vi "Score Gear Auto.vi"(8 "Command Info in":T1, 9 "speed of backing up":dbl=0.3 format="%#_13g", 10 "Seconds of backing up":dbl=2.0 format="%#_13g") -> (0 "Command Info Out":T1)   [LabVIEW 2016]
uses:
  <vilib>/Rock Robotics/WPI/Framework/Command Status Info.ctl
  <vilib>/Rock Robotics/WPI/Framework/Completion Status.ctl
  <vilib>/Rock Robotics/WPI/Framework/Completion Notifier.ctl
  <vilib>/Rock Robotics/WPI/Solenoid/WPI_SolenoidValue.ctl
  <vilib>/Rock Robotics/WPI/Solenoid/WPI_SolenoidSetEnum.vi
panel:
  in  "Seconds to wait 2":dbl=0.25 format="%#_13g"
  in  "Seconds to wait":dbl=0.15 format="%#_13g"
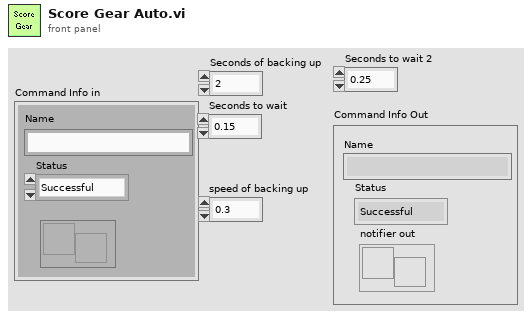
[diagram p1: front panel]
types:
  T1 = typedef "Command Status Info.ctl" = cluster{"Name":string, "Status":T2, "notifier out":T3}
  T2 = typedef "Completion Status.ctl" = enum16{"Successful", "Aborted", "Incomplete"}
  T3 = typedef "Completion Notifier.ctl" = refnum<notifier>
  T4 = typedef "WPI_SolenoidValue.ctl" = enum16{"Off", "On", "Forward", "Reverse"}
  T5 = typedef "WPI_MotorControlDeviceRef.ctl" = cluster{"DeviceStatus":errorcluster, "Type":T6, "PWM":cluster{"PWM Channel":T7, "DeadBand":T8}, "CAN":cluster{"Device Number":u8, "SetOutput VI Ref":variant, "GetOutput VI Ref":variant, "Enable VI Ref":variant, "Disable VI Ref":variant, "Data":variant}, "Invert":bool}
  T6 = typedef "WPI_MotorControlType.ctl" = enum16{"PWM", "CAN"}
  T7 = typedef "FPGA_DIOPWMChannel.ctl" = enum8{"PWM 0", "PWM 1", "PWM 2", "PWM 3", "PWM 4", "PWM 5", "PWM 6", "PWM 7", "PWM 8", "PWM 9", "PWM MXP 0", "PWM MXP 1", "PWM MXP 2", "PWM MXP 3", "PWM MXP 4", "PWM MXP 5", "PWM MXP 6", "PWM MXP 7", "PWM MXP 8", "PWM MXP 9", "Invalid"}
  T8 = typedef "WPI_PWMDeadband.ctl" = cluster{"Name":string, "maxPositivePwm":i32, "minPositivePwm":i32, "centerPwm":i32, "maxNegativePwm":i32, "minNegativePwm":i32, "angularRange":u16}
  T9 = typedef "WPI_SolenoidDevRef.ctl" = cluster{"DevStatus":errorcluster, "Pneumatics Control Module":u8, "Forward Solenoid Channel":T10, "Reverse Solenoid Channel":T10}
  T10 = typedef "WPI_SolenoidChannel.ctl" = enum8{"Solenoid 0", "Solenoid 1", "Solenoid 2", "Solenoid 3", "Solenoid 4", "Solenoid 5", "Solenoid 6", "Solenoid 7", "Invalid"}
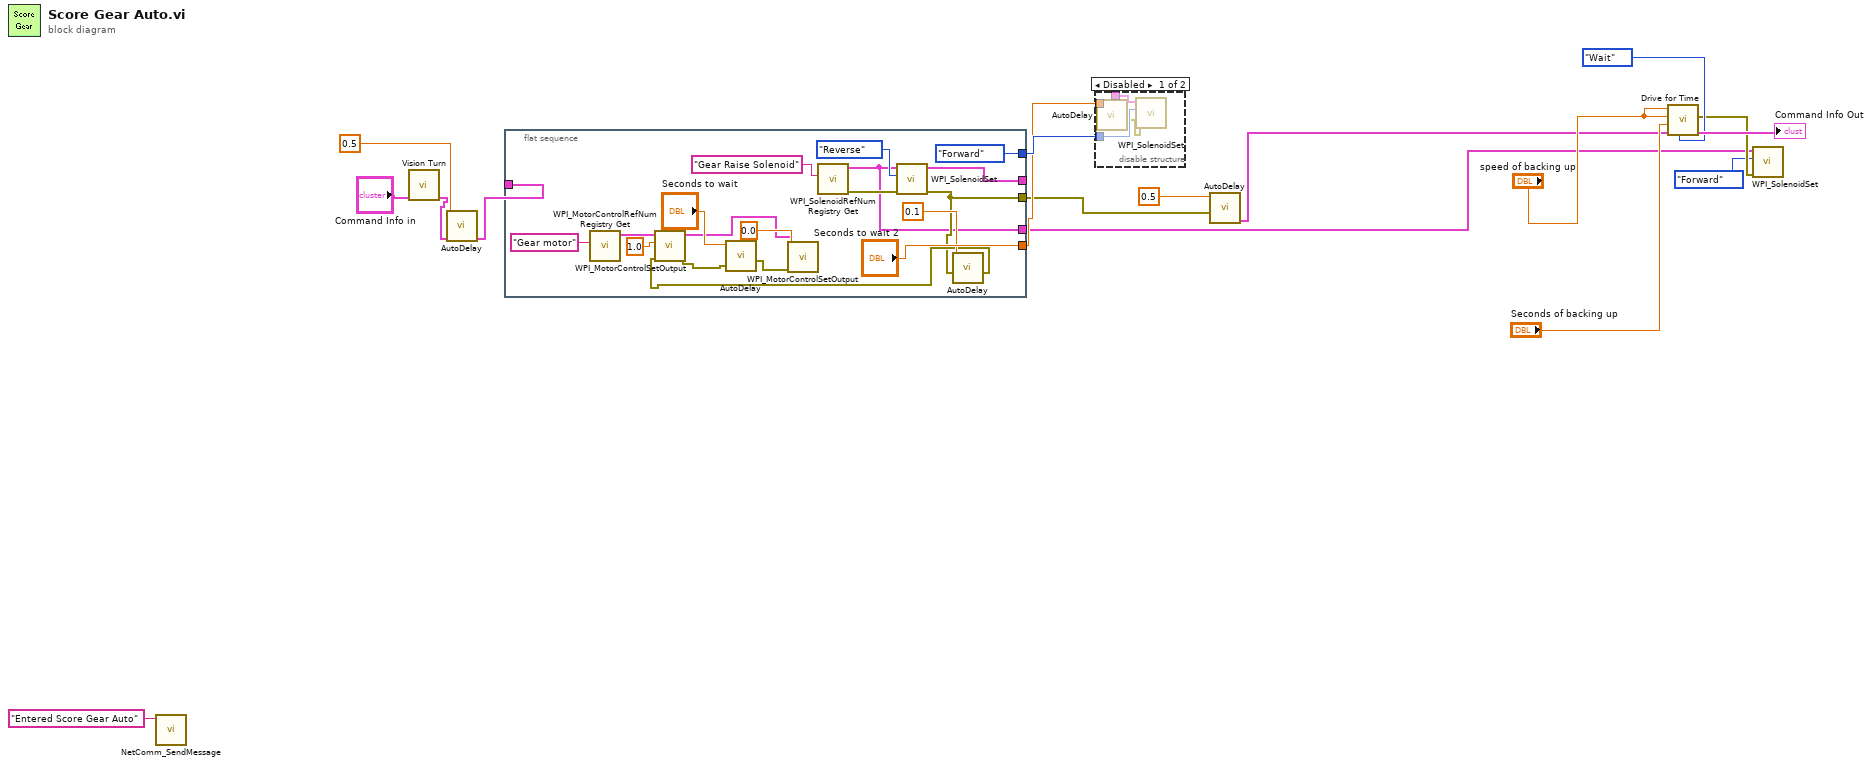
[diagram p0: block diagram]
diagram:
  n1 = call <vilib>:"NetComm_SendMessage.vi"("Message"="Entered Score Gear Auto") -> ()  [unwired: 11 in]
  n2 = call "Vision Turn.vi"("Command Info In"="Command Info in") -> ("Command Info Out"=w11:T1)  [unwired: 10 in]
  n3 = call "AutoDelay.vi"("Command Info In"=w11, "Seconds to wait"=0.5) -> ("Command Info Out"=w10:T1)  [unwired: 8 in, 1 out]
  n4 = flat-sequence {
    tunnel: w10 -> [_]
    tunnel: [w24] -> _
    tunnel: [WPI_SolenoidValue."Forward" ("Value")] -> w8
    tunnel: ["Seconds to wait 2"] -> w7
    tunnel: [w19] -> w5
    tunnel: [w18] -> w2
    frame #0 {
      n5 = call <vilib>:"WPI_MotorControlRefNum Registry Get.vi"("refnum name"="Gear motor") -> ("MotorControlDevRef"=w30:T5)  [unwired: 9 in, 1 out]
      n6 = call <vilib>:"WPI_SolenoidRefNum Registry Get.vi"("refnum name"="Gear Raise Solenoid") -> ("error out"=w34:errorcluster, "SolenoidDevRef"=w18:T9)  [unwired: 9 in]
      n7 = call-poly <vilib>:"WPI_SolenoidSet.vi"("error in (no error)"=w34, "Value"=WPI_SolenoidValue."Reverse", "SolenoidDevRef"=w18) -> ("error out"=w19:errorcluster, "SolenoidDevRef"=w24:T9)  [unwired: 7 in]
      n8 = call "AutoDelay.vi"("error in (no error)"=w19, "Seconds to wait"=0.1) -> ("error out (no error)"=w20:errorcluster)  [unwired: 8 in, 1 out]
      n9 = call <vilib>:"WPI_MotorControlSetOutput.vi"("error in (no error)"=w20, "Output"=1.0, "MotorControlDevRef"=w30) -> ("error out"=w28:errorcluster, "MotorControlDevRef"=w25:T5)  [unwired: 6 in, 1 out]
      n10 = call "AutoDelay.vi"("error in (no error)"=w28, "Seconds to wait"="Seconds to wait") -> ("error out (no error)"=w27:errorcluster)  [unwired: 8 in, 1 out]
      n11 = call <vilib>:"WPI_MotorControlSetOutput.vi"("error in (no error)"=w27, "Output"=0.0, "MotorControlDevRef"=w25) -> ()  [unwired: 6 in, 3 out]
    }
  }
  n12 = disable-structure shown="Disabled" {
    disable-tunnel: _ -> [w39 _]
    disable-tunnel: w8 -> [w38 _]
    disable-tunnel: w7 -> [w36 _]
    frame Disabled {
      n13 = call "AutoDelay.vi"("Seconds to wait"=w36) -> ("error out (no error)"=w37:errorcluster)  [unwired: 9 in, 1 out]
      n14 = call-poly <vilib>:"WPI_SolenoidSet.vi"("error in (no error)"=w37, "Value"=w38, "SolenoidDevRef"=w39) -> ()  [unwired: 7 in, 2 out]
    }
    frame Enabled {
    }
  }
  n15 = call "AutoDelay.vi"("error in (no error)"=w5, "Seconds to wait"=0.5) -> ("Command Info Out"=w4:T1)  [unwired: 8 in, 1 out]
  n16 = call "Drive for Time.vi"("Synchronization"=enum16{"Start", "Wait"}."Wait" ("Synchronication"), "Command Info In"=w4, "Seconds"="Seconds of backing up", "Right Speed"="speed of backing up", "Left Speed"="speed of backing up") -> ("Command Info Out"=→"Command Info Out":T1, "error out"=w3:errorcluster)  [unwired: 4 in, 1 out]
  n17 = call-poly <vilib>:"WPI_SolenoidSet.vi"("error in (no error)"=w3, "Value"=WPI_SolenoidValue."Forward", "SolenoidDevRef"=w2) -> ()  [unwired: 7 in, 2 out]
